vi "App - analyze RUS V6.vi"() -> ()   [LabVIEW 2021] (continued)
"file format"=enum."binary", "power(V)"=2.1, "Magn Field(T) "=0.0}, {"temperature"=14.639, "temperature str"="14.63900", "file path"=path "D:/Data/Ultrasound/LSCO/LSCO22__130814c/5_Cooling_2nd_try/September_2014/091814/14.63900K_500_2500_2.10000V_0.00000T_Sep18-2014__09-59-22_001_091814.bin", "last mod"=timestamp(3493893562 s since 1904-01-01), "file name str"="D:\\Data\\Ultrasound\\LSCO\\LSCO22__130814c\\5_Cooling_2nd_try\\September_2014\\091814\\14.63900K_500_2500_2.10000V_0.00000T_Sep18-2014__09-59-22_001_091814.bin", "mod time(min)"=58231559.36666667, "file format"=enum."binary", "power(V)"=2.1, "Magn Field(T) "=0.0}, {"temperature"=14.64, "temperature str"="14.64000", "file path"=path "D:/Data/Ultrasound/LSCO/LSCO22__130814c/5_Cooling_2nd_try/September_2014/091814/14.64000K_500_2500_2.10000V_0.00000T_Sep18-2014__10-00-41_001_091814.bin", "last mod"=timestamp(3493893641 s since 1904-01-01), "file name str"="D:\\Data\\Ultrasound\\LSCO\\LSCO22__130814c\\5_Cooling_2nd_try\\September_2014\\091814\\14.64000K_500_2500_2.10000V_0.00000T_Sep18-2014__10-00-41_001_091814.bin", "mod time(min)"=58231560.68333333, "file format"=enum."binary", "power(V)"=2.1, "Magn Field(T) "=0.0}, {"temperature"=14.641, "temperature str"="14.64100", "file path"=path "D:/Data/Ultrasound/LSCO/LSCO22__130814c/5_Cooling_2nd_try/September_2014/091814/14.64100K_500_2500_2.10000V_0.00000T_Sep18-2014__10-02-01_001_091814.bin", "last mod"=timestamp(3493893721 s since 1904-01-01), "file name str"="D:\\Data\\Ultrasound\\LSCO\\LSCO22__130814c\\5_Cooling_2nd_try\\September_2014\\091814\\14.64100K_500_2500_2.10000V_0.00000T_Sep18-2014__10-02-01_001_091814.bin", "mod time(min)"=58231562.016666666, "file format"=enum."binary", "power(V)"=2.1, "Magn Field(T) "=0.0}, {"temperature"=14.644, "temperature str"="14.64400", "file path"=path "D:/Data/Ultrasound/LSCO/LSCO22__130814c/5_Cooling_2nd_try/September_2014/091814/14.64400K_500_2500_2.10000V_0.00000T_Sep18-2014__10-03-20_001_091814.bin", "last mod"=timestamp(3493893800 s since 1904-01-01), "file name str"="D:\\Data\\Ultrasound\\LSCO\\LSCO22__130814c\\5_Cooling_2nd_try\\September_2014\\091814\\14.64400K_500_2500_2.10000V_0.00000T_Sep18-2014__10-03-20_001_091814.bin", "mod time(min)"=58231563.333333336, "file format"=enum."binary", "power(V)"=2.1, "Magn Field(T) "=0.0}, {"temperature"=14.65, "temperature str"="14.65000", "file path"=path "D:/Data/Ultrasound/LSCO/LSCO22__130814c/5_Cooling_2nd_try/September_2014/091814/14.65000K_500_2500_2.10000V_0.00000T_Sep18-2014__10-04-39_001_091814.bin", "last mod"=timestamp(3493893879 s since 1904-01-01), "file name str"="D:\\Data\\Ultrasound\\LSCO\\LSCO22__130814c\\5_Cooling_2nd_try\\September_2014\\091814\\14.65000K_500_2500_2.10000V_0.00000T_Sep18-2014__10-04-39_001_091814.bin", "mod time(min)"=58231564.65, "file format"=enum."binary", "power(V)"=2.1, "Magn Field(T) "=0.0}, {"temperature"=14.65, "temperature str"="14.65000", "file path"=path "D:/Data/Ultrasound/LSCO/LSCO22__130814c/5_Cooling_2nd_try/September_2014/091814/14.65000K_500_2500_2.10000V_0.00000T_Sep18-2014__10-05-59_001_091814.bin", "last mod"=timestamp(3493893959 s since 1904-01-01), "file name str"="D:\\Data\\Ultrasound\\LSCO\\LSCO22__130814c\\5_Cooling_2nd_try\\September_2014\\091814\\14.65000K_500_2500_2.10000V_0.00000T_Sep18-2014__10-05-59_001_091814.bin", "mod time(min)"=58231565.983333334, "file format"=enum."binary", "power(V)"=2.1, "Magn Field(T) "=0.0}, {"temperature"=14.654, "temperature str"="14.65400", "file path"=path "D:/Data/Ultrasound/LSCO/LSCO22__130814c/5_Cooling_2nd_try/September_2014/091814/14.65400K_500_2500_2.10000V_0.00000T_Sep18-2014__10-07-18_001_091814.bin", "last mod"=timestamp(3493894038 s since 1904-01-01), "file name str"="D:\\Data\\Ultrasound\\LSCO\\LSCO22__130814c\\5_Cooling_2nd_try\\September_2014\\091814\\14.65400K_500_2500_2.10000V_0.00000T_Sep18-2014__10-07-18_001_091814.bin", "mod time(min)"=58231567.3, "file format"=enum."binary", "power(V)"=2.1, "Magn Field(T) "=0.0}, {"temperature"=14.654, "temperature str"="14.65400", "file path"=path "D:/Data/Ultrasound/LSCO/LSCO22__130814c/5_Cooling_2nd_try/September_2014/091814/14.65400K_500_2500_2.10000V_0.00000T_Sep18-2014__10-08-38_001_091814.bin", "last mod"=timestamp(3493894118 s since 1904-01-01), "file name str"="D:\\Data\\Ultrasound\\LSCO\\LSCO22__130814c\\5_Cooling_2nd_try\\September_2014\\091814\\14.65400K_500_2500_2.10000V_0.00000T_Sep18-2014__10-08-38_001_091814.bin", "mod time(min)"=58231568.63333333, "file format"=enum."binary", "power(V)"=2.1, "Magn Field(T) "=0.0}, {"temperature"=14.657, "temperature str"="14.65700", "file path"=path "D:/Data/Ultrasound/LSCO/LSCO22__130814c/5_Cooling_2nd_try/September_2014/091814/14.65700K_500_2500_2.10000V_0.00000T_Sep18-2014__10-09-57_001_091814.bin", "last mod"=timestamp(3493894197 s since 1904-01-01), "file name str"="D:\\Data\\Ultrasound\\LSCO\\LSCO22__130814c\\5_Cooling_2nd_try\\September_2014\\091814\\14.65700K_500_2500_2.10000V_0.00000T_Sep18-2014__10-09-57_001_091814.bin", "mod time(min)"=58231569.95, "file format"=enum."binary", "power(V)"=2.1, "Magn Field(T) "=0.0}, {"temperature"=14.659, "temperature str"="14.65900", "file path"=path "D:/Data/Ultrasound/LSCO/LSCO22__130814c/5_Cooling_2nd_try/September_2014/091814/14.65900K_500_2500_2.10000V_0.00000T_Sep18-2014__10-11-16_001_091814.bin", "last mod"=timestamp(3493894276 s since 1904-01-01), "file name str"="D:\\Data\\Ultrasound\\LSCO\\LSCO22__130814c\\5_Cooling_2nd_try\\September_2014\\091814\\14.65900K_500_2500_2.10000V_0.00000T_Sep18-2014__10-11-16_001_091814.bin", "mod time(min)"=58231571.266666666, "file format"=enum."binary", "power(V)"=2.1, "Magn Field(T) "=0.0}, {"temperature"=14.66, "temperature str"="14.66000", "file path"=path "D:/Data/Ultrasound/LSCO/LSCO22__130814c/5_Cooling_2nd_try/September_2014/091814/14.66000K_500_2500_2.10000V_0.00000T_Sep18-2014__10-12-36_001_091814.bin", "last mod"=timestamp(3493894356 s since 1904-01-01), "file name str"="D:\\Data\\Ultrasound\\LSCO\\LSCO22__130814c\\5_Cooling_2nd_try\\September_2014\\091814\\14.66000K_500_2500_2.10000V_0.00000T_Sep18-2014__10-12-36_001_091814.bin", "mod time(min)"=58231572.6, "file format"=enum."binary", "power(V)"=2.1, "Magn Field(T) "=0.0}, {"temperature"=14.661, "temperature str"="14.66100", "file path"=path "D:/Data/Ultrasound/LSCO/LSCO22__130814c/5_Cooling_2nd_try/September_2014/091814/14.66100K_500_2500_2.10000V_0.00000T_Sep18-2014__10-13-55_001_091814.bin", "last mod"=timestamp(3493894435 s since 1904-01-01), "file name str"="D:\\Data\\Ultrasound\\LSCO\\LSCO22__130814c\\5_Cooling_2nd_try\\September_2014\\091814\\14.66100K_500_2500_2.10000V_0.00000T_Sep18-2014__10-13-55_001_091814.bin", "mod time(min)"=58231573.916666664, "file format"=enum."binary", "power(V)"=2.1, "Magn Field(T) "=0.0}, {"temperature"=14.664, "temperature str"="14.66400", "file path"=path "D:/Data/Ultrasound/LSCO/LSCO22__130814c/5_Cooling_2nd_try/September_2014/091814/14.66400K_500_2500_2.10000V_0.00000T_Sep18-2014__10-15-14_001_091814.bin", "last mod"=timestamp(3493894514 s since 1904-01-01), "file name str"="D:\\Data\\Ultrasound\\LSCO\\LSCO22__130814c\\5_Cooling_2nd_try\\September_2014\\091814\\14.66400K_500_2500_2.10000V_0.00000T_Sep18-2014__10-15-14_001_091814.bin", "mod time(min)"=58231575.233333334, "file format"=enum."binary", "power(V)"=2.1, "Magn Field(T) "=0.0}, {"temperature"=14.668, "temperature str"="14.66800", "file path"=path "D:/Data/Ultrasound/LSCO/LSCO22__130814c/5_Cooling_2nd_try/September_2014/091814/14.66800K_500_2500_2.10000V_0.00000T_Sep18-2014__10-16-34_001_091814.bin", "last mod"=timestamp(3493894594 s since 1904-01-01), "file name str"="D:\\Data\\Ultrasound\\LSCO\\LSCO22__130814c\\5_Cooling_2nd_try\\September_2014\\091814\\14.66800K_500_2500_2.10000V_0.00000T_Sep18-2014__10-16-34_001_091814.bin", "mod time(min)"=58231576.56666667, "file format"=enum."binary", "power(V)"=2.1, "Magn Field(T) "=0.0}, {"temperature"=14.669, "temperature str"="14.66900", "file path"=path "D:/Data/Ultrasound/LSCO/LSCO22__130814c/5_Cooling_2nd_try/September_2014/091814/14.66900K_500_2500_2.10000V_0.00000T_Sep18-2014__10-17-53_001_091814.bin", "last mod"=timestamp(3493894673 s since 1904-01-01), "file name str"="D:\\Data\\Ultrasound\\LSCO\\LSCO22__130814c\\5_Cooling_2nd_try\\September_2014\\091814\\14.66900K_500_2500_2.10000V_0.00000T_Sep18-2014__10-17-53_001_091814.bin", "mod time(min)"=58231577.88333333, "file format"=enum."binary", "power(V)"=2.1, "Magn Field(T) "=0.0}, {"temperature"=14.673, "temperature str"="14.67300", "file path"=path "D:/Data/Ultrasound/LSCO/LSCO22__130814c/5_Cooling_2nd_try/September_2014/091814/14.67300K_500_2500_2.10000V_0.00000T_Sep18-2014__10-19-13_001_091814.bin", "last mod"=timestamp(3493894753 s since 1904-01-01), "file name str"="D:\\Data\\Ultrasound\\LSCO\\LSCO22__130814c\\5_Cooling_2nd_try\\September_2014\\091814\\14.67300K_500_2500_2.10000V_0.00000T_Sep18-2014__10-19-13_001_091814.bin", "mod time(min)"=58231579.21666667, "file format"=enum."binary", "power(V)"=2.1, "Magn Field(T) "=0.0}, {"temperature"=14.673, "temperature str"="14.67300", "file path"=path "D:/Data/Ultrasound/LSCO/LSCO22__130814c/5_Cooling_2nd_try/September_2014/091814/14.67300K_500_2500_2.10000V_0.00000T_Sep18-2014__10-20-32_001_091814.bin", "last mod"=timestamp(3493894832 s since 1904-01-01), "file name str"="D:\\Data\\Ultrasound\\LSCO\\LSCO22__130814c\\5_Cooling_2nd_try\\September_2014\\091814\\14.67300K_500_2500_2.10000V_0.00000T_Sep18-2014__10-20-32_001_091814.bin", "mod time(min)"=58231580.53333333, "file format"=enum."binary", "power(V)"=2.1, "Magn Field(T) "=0.0}, {"temperature"=14.673, "temperature str"="14.67300", "file path"=path "D:/Data/Ultrasound/LSCO/LSCO22__130814c/5_Cooling_2nd_try/September_2014/091814/14.67300K_500_2500_2.10000V_0.00000T_Sep18-2014__10-21-51_001_091814.bin", "last mod"=timestamp(3493894911 s since 1904-01-01), "file name str"="D:\\Data\\Ultrasound\\LSCO\\LSCO22__130814c\\5_Cooling_2nd_try\\September_2014\\091814\\14.67300K_500_2500_2.10000V_0.00000T_Sep18-2014__10-21-51_001_091814.bin", "mod time(min)"=58231581.85, "file format"=enum."binary", "power(V)"=2.1, "Magn Field(T) "=0.0}, {"temperature"=14.676, "temperature str"="14.67600", "file path"=path "D:/Data/Ultrasound/LSCO/LSCO22__130814c/5_Cooling_2nd_try/September_2014/091814/14.67600K_500_2500_2.10000V_0.00000T_Sep18-2014__10-23-11_001_091814.bin", "last mod"=timestamp(3493894991 s since 1904-01-01), "file name str"="D:\\Data\\Ultrasound\\LSCO\\LSCO22__130814c\\5_Cooling_2nd_try\\September_2014\\091814\\14.67600K_500_2500_2.10000V_0.00000T_Sep18-2014__10-23-11_001_091814.bin", "mod time(min)"=58231583.18333333, "file format"=enum."binary", "power(V)"=2.1, "Magn Field(T) "=0.0}, {"temperature"=14.678, "temperature str"="14.67800", "file path"=path "D:/Data/Ultrasound/LSCO/LSCO22__130814c/5_Cooling_2nd_try/September_2014/091814/14.67800K_500_2500_2.10000V_0.00000T_Sep18-2014__10-24-30_001_091814.bin", "last mod"=timestamp(3493895070 s since 1904-01-01), "file name str"="D:\\Data\\Ultrasound\\LSCO\\LSCO22__130814c\\5_Cooling_2nd_try\\September_2014\\091814\\14.67800K_500_2500_2.10000V_0.00000T_Sep18-2014__10-24-30_001_091814.bin", "mod time(min)"=58231584.5, "file format"=enum."binary", "power(V)"=2.1, "Magn Field(T) "=0.0}, {"temperature"=14.678, "temperature str"="14.67800", "file path"=path "D:/Data/Ultrasound/LSCO/LSCO22__130814c/5_Cooling_2nd_try/September_2014/091814/14.67800K_500_2500_2.10000V_0.00000T_Sep18-2014__10-25-49_001_091814.bin", "last mod"=timestamp(3493895149 s since 1904-01-01), "file name str"="D:\\Data\\Ultrasound\\LSCO\\LSCO22__130814c\\5_Cooling_2nd_try\\September_2014\\091814\\14.67800K_500_2500_2.10000V_0.00000T_Sep18-2014__10-25-49_001_091814.bin", "mod time(min)"=58231585.81666667, "file format"=enum."binary", "power(V)"=2.1, "Magn Field(T) "=0.0}, {"temperature"=14.681, "temperature str"="14.68100", "file path"=path "D:/Data/Ultrasound/LSCO/LSCO22__130814c/5_Cooling_2nd_try/September_2014/091814/14.68100K_500_2500_2.10000V_0.00000T_Sep18-2014__10-27-09_001_091814.bin", "last mod"=timestamp(3493895229 s since 1904-01-01), "file name str"="D:\\Data\\Ultrasound\\LSCO\\LSCO22__130814c\\5_Cooling_2nd_try\\September_2014\\091814\\14.68100K_500_2500_2.10000V_0.00000T_Sep18-2014__10-27-09_001_091814.bin", "mod time(min)"=58231587.15, "file format"=enum."binary", "power(V)"=2.1, "Magn Field(T) "=0.0}, {"temperature"=14.682, "temperature str"="14.68200", "file path"=path "D:/Data/Ultrasound/LSCO/LSCO22__130814c/5_Cooling_2nd_try/September_2014/091814/14.68200K_500_2500_2.10000V_0.00000T_Sep18-2014__10-28-28_001_091814.bin", "last mod"=timestamp(3493895308 s since 1904-01-01), "file name str"="D:\\Data\\Ultrasound\\LSCO\\LSCO22__130814c\\5_Cooling_2nd_try\\September_2014\\091814\\14.68200K_500_2500_2.10000V_0.00000T_Sep18-2014__10-28-28_001_091814.bin", "mod time(min)"=58231588.46666667, "file format"=enum."binary", "power(V)"=2.1, "Magn Field(T) "=0.0}, {"temperature"=14.685, "temperature str"="14.68500", "file path"=path "D:/Data/Ultrasound/LSCO/LSCO22__130814c/5_Cooling_2nd_try/September_2014/091814/14.68500K_500_2500_2.10000V_0.00000T_Sep18-2014__10-29-48_001_091814.bin", "last mod"=timestamp(3493895388 s since 1904-01-01), "file name str"="D:\\Data\\Ultrasound\\LSCO\\LSCO22__130814c\\5_Cooling_2nd_try\\September_2014\\091814\\14.68500K_500_2500_2.10000V_0.00000T_Sep18-2014__10-29-48_001_091814.bin", "mod time(min)"=58231589.8, "file format"=enum."binary", "power(V)"=2.1, "Magn Field(T) "=0.0}, {"temperature"=14.689, "temperature str"="14.68900", "file path"=path "D:/Data/Ultrasound/LSCO/LSCO22__130814c/5_Cooling_2nd_try/September_2014/091814/14.68900K_500_2500_2.10000V_0.00000T_Sep18-2014__10-31-07_001_091814.bin", "last mod"=timestamp(3493895467 s since 1904-01-01), "file name str"="D:\\Data\\Ultrasound\\LSCO\\LSCO22__130814c\\5_Cooling_2nd_try\\September_2014\\091814\\14.68900K_500_2500_2.10000V_0.00000T_Sep18-2014__10-31-07_001_091814.bin", "mod time(min)"=58231591.11666667, "file format"=enum."binary", "power(V)"=2.1, "Magn Field(T) "=0.0}, {"temperature"=14.687, "temperature str"="14.68700", "file path"=path "D:/Data/Ultrasound/LSCO/LSCO22__130814c/5_Cooling_2nd_try/September_2014/091814/14.68700K_500_2500_2.10000V_0.00000T_Sep18-2014__10-32-26_001_091814.bin", "last mod"=timestamp(3493895546 s since 1904-01-01), "file name str"="D:\\Data\\Ultrasound\\LSCO\\LSCO22__130814c\\5_Cooling_2nd_try\\September_2014\\091814\\14.68700K_500_2500_2.10000V_0.00000T_Sep18-2014__10-32-26_001_091814.bin", "mod time(min)"=58231592.43333333, "file format"=enum."binary", "power(V)"=2.1, "Magn Field(T) "=0.0}, {"temperature"=14.688, "temperature str"="14.68800", "file path"=path "D:/Data/Ultrasound/LSCO/LSCO22__130814c/5_Cooling_2nd_try/September_2014/091814/14.68800K_500_2500_2.10000V_0.00000T_Sep18-2014__10-33-46_001_091814.bin", "last mod"=timestamp(3493895626 s since 1904-01-01), "file name str"="D:\\Data\\Ultrasound\\LSCO\\LSCO22__130814c\\5_Cooling_2nd_try\\September_2014\\091814\\14.68800K_500_2500_2.10000V_0.00000T_Sep18-2014__10-33-46_001_091814.bin", "mod time(min)"=58231593.766666666, "file format"=enum."binary", "power(V)"=2.1, "Magn Field(T) "=0.0}, {"temperature"=14.693, "temperature str"="14.69300", "file path"=path "D:/Data/Ultrasound/LSCO/LSCO22__130814c/5_Cooling_2nd_try/September_2014/091814/14.69300K_500_2500_2.10000V_0.00000T_Sep18-2014__10-35-05_001_091814.bin", "last mod"=timestamp(3493895705 s since 1904-01-01), "file name str"="D:\\Data\\Ultrasound\\LSCO\\LSCO22__130814c\\5_Cooling_2nd_try\\September_2014\\091814\\14.69300K_500_2500_2.10000V_0.00000T_Sep18-2014__10-35-05_001_091814.bin", "mod time(min)"=58231595.083333336, "file format"=enum."binary", "power(V)"=2.1, "Magn Field(T) "=0.0}, {"temperature"=14.693, "temperature str"="14.69300", "file path"=path "D:/Data/Ultrasound/LSCO/LSCO22__130814c/5_Cooling_2nd_try/September_2014/091814/14.69300K_500_2500_2.10000V_0.00000T_Sep18-2014__10-36-24_001_091814.bin", "last mod"=timestamp(3493895784 s since 1904-01-01), "file name str"="D:\\Data\\Ultrasound\\LSCO\\LSCO22__130814c\\5_Cooling_2nd_try\\September_2014\\091814\\14.69300K_500_2500_2.10000V_0.00000T_Sep18-2014__10-36-24_001_091814.bin", "mod time(min)"=58231596.4, "file format"=enum."binary", "power(V)"=2.1, "Magn Field(T) "=0.0}, {"temperature"=14.696, "temperature str"="14.69600", "file path"=path "D:/Data/Ultrasound/LSCO/LSCO22__130814c/5_Cooling_2nd_try/September_2014/091814/14.69600K_500_2500_2.10000V_0.00000T_Sep18-2014__10-37-44_001_091814.bin", "last mod"=timestamp(3493895864 s since 1904-01-01), "file name str"="D:\\Data\\Ultrasound\\LSCO\\LSCO22__130814c\\5_Cooling_2nd_try\\September_2014\\091814\\14.69600K_500_2500_2.10000V_0.00000T_Sep18-2014__10-37-44_001_091814.bin", "mod time(min)"=58231597.733333334, "file format"=enum."binary", "power(V)"=2.1, "Magn Field(T) "=0.0}, {"temperature"=14.697, "temperature str"="14.69700", "file path"=path "D:/Data/Ultrasound/LSCO/LSCO22__130814c/5_Cooling_2nd_try/September_2014/091814/14.69700K_500_2500_2.10000V_0.00000T_Sep18-2014__10-39-03_001_091814.bin", "last mod"=timestamp(3493895943 s since 1904-01-01), "file name str"="D:\\Data\\Ultrasound\\LSCO\\LSCO22__130814c\\5_Cooling_2nd_try\\September_2014\\091814\\14.69700K_500_2500_2.10000V_0.00000T_Sep18-2014__10-39-03_001_091814.bin", "mod time(min)"=58231599.05, "file format"=enum."binary", "power(V)"=2.1, "Magn Field(T) "=0.0}, {"temperature"=14.697, "temperature str"="14.69700", "file path"=path "D:/Data/Ultrasound/LSCO/LSCO22__130814c/5_Cooling_2nd_try/September_2014/091814/14.69700K_500_2500_2.10000V_0.00000T_Sep18-2014__10-40-23_001_091814.bin", "last mod"=timestamp(3493896023 s since 1904-01-01), "file name str"="D:\\Data\\Ultrasound\\LSCO\\LSCO22__130814c\\5_Cooling_2nd_try\\September_2014\\091814\\14.69700K_500_2500_2.10000V_0.00000T_Sep18-2014__10-40-23_001_091814.bin", "mod time(min)"=58231600.38333333, "file format"=enum."binary", "power(V)"=2.1, "Magn Field(T) "=0.0}, {"temperature"=14.699, "temperature str"="14.69900", "file path"=path "D:/Data/Ultrasound/LSCO/LSCO22__130814c/5_Cooling_2nd_try/September_2014/091814/14.69900K_500_2500_2.10000V_0.00000T_Sep18-2014__10-41-42_001_091814.bin", "last mod"=timestamp(3493896102 s since 1904-01-01), "file name str"="D:\\Data\\Ultrasound\\LSCO\\LSCO22__130814c\\5_Cooling_2nd_try\\September_2014\\091814\\14.69900K_500_2500_2.10000V_0.00000T_Sep18-2014__10-41-42_001_091814.bin", "mod time(min)"=58231601.7, "file format"=enum."binary", "power(V)"=2.1, "Magn Field(T) "=0.0}, {"temperature"=14.702, "temperature str"="14.70200", "file path"=path "D:/Data/Ultrasound/LSCO/LSCO22__130814c/5_Cooling_2nd_try/September_2014/091814/14.70200K_500_2500_2.10000V_0.00000T_Sep18-2014__10-43-01_001_091814.bin", "last mod"=timestamp(3493896181 s since 1904-01-01), "file name str"="D:\\Data\\Ultrasound\\LSCO\\LSCO22__130814c\\5_Cooling_2nd_try\\September_2014\\091814\\14.70200K_500_2500_2.10000V_0.00000T_Sep18-2014__10-43-01_001_091814.bin", "mod time(min)"=58231603.016666666, "file format"=enum."binary", "power(V)"=2.1, "Magn Field(T) "=0.0}, {"temperature"=14.706, "temperature str"="14.70600", "file path"=path "D:/Data/Ultrasound/LSCO/LSCO22__130814c/5_Cooling_2nd_try/September_2014/091814/14.70600K_500_2500_2.10000V_0.00000T_Sep18-2014__10-44-21_001_091814.bin", "last mod"=timestamp(3493896261 s since 1904-01-01), "file name str"="D:\\Data\\Ultrasound\\LSCO\\LSCO22__130814c\\5_Cooling_2nd_try\\September_2014\\091814\\14.70600K_500_2500_2.10000V_0.00000T_Sep18-2014__10-44-21_001_091814.bin", "mod time(min)"=58231604.35, "file format"=enum."binary", "power(V)"=2.1, "Magn Field(T) "=0.0}, {"temperature"=14.708, "temperature str"="14.70800", "file path"=path "D:/Data/Ultrasound/LSCO/LSCO22__130814c/5_Cooling_2nd_try/September_2014/091814/14.70800K_500_2500_2.10000V_0.00000T_Sep18-2014__10-45-40_001_091814.bin", "last mod"=timestamp(3493896340 s since 1904-01-01), "file name str"="D:\\Data\\Ultrasound\\LSCO\\LSCO22__130814c\\5_Cooling_2nd_try\\September_2014\\091814\\14.70800K_500_2500_2.10000V_0.00000T_Sep18-2014__10-45-40_001_091814.bin", "mod time(min)"=58231605.666666664, "file format"=enum."binary", "power(V)"=2.1, "Magn Field(T) "=0.0}, {"temperature"=14.703, "temperature str"="14.70300", "file path"=path "D:/Data/Ultrasound/LSCO/LSCO22__130814c/5_Cooling_2nd_try/September_2014/091814/14.70300K_500_2500_2.10000V_0.00000T_Sep18-2014__10-46-59_001_091814.bin", "last mod"=timestamp(3493896419 s since 1904-01-01), "file name str"="D:\\Data\\Ultrasound\\LSCO\\LSCO22__130814c\\5_Cooling_2nd_try\\September_2014\\091814\\14.70300K_500_2500_2.10000V_0.00000T_Sep18-2014__10-46-59_001_091814.bin", "mod time(min)"=58231606.983333334, "file format"=enum."binary", "power(V)"=2.1, "Magn Field(T) "=0.0}, {"temperature"=14.705, "temperature str"="14.70500", "file path"=path "D:/Data/Ultrasound/LSCO/LSCO22__130814c/5_Cooling_2nd_try/September_2014/091814/14.70500K_500_2500_2.10000V_0.00000T_Sep18-2014__10-48-19_001_091814.bin", "last mod"=timestamp(3493896499 s since 1904-01-01), "file name str"="D:\\Data\\Ultrasound\\LSCO\\LSCO22__130814c\\5_Cooling_2nd_try\\September_2014\\091814\\14.70500K_500_2500_2.10000V_0.00000T_Sep18-2014__10-48-19_001_091814.bin", "mod time(min)"=58231608.31666667, "file format"=enum."binary", "power(V)"=2.1, "Magn Field(T) "=0.0}, {"temperature"=14.708, "temperature str"="14.70800", "file path"=path "D:/Data/Ultrasound/LSCO/LSCO22__130814c/5_Cooling_2nd_try/September_2014/091814/14.70800K_500_2500_2.10000V_0.00000T_Sep18-2014__10-49-38_001_091814.bin", "last mod"=timestamp(3493896578 s since 1904-01-01), "file name str"="D:\\Data\\Ultrasound\\LSCO\\LSCO22__130814c\\5_Cooling_2nd_try\\September_2014\\091814\\14.70800K_500_2500_2.10000V_0.00000T_Sep18-2014__10-49-38_001_091814.bin", "mod time(min)"=58231609.63333333, "file format"=enum."binary", "power(V)"=2.1, "Magn Field(T) "=0.0}, {"temperature"=14.709, "temperature str"="14.70900", "file path"=path "D:/Data/Ultrasound/LSCO/LSCO22__130814c/5_Cooling_2nd_try/September_2014/091814/14.70900K_500_2500_2.10000V_0.00000T_Sep18-2014__10-50-58_001_091814.bin", "last mod"=timestamp(3493896658 s since 1904-01-01), "file name str"="D:\\Data\\Ultrasound\\LSCO\\LSCO22__130814c\\5_Cooling_2nd_try\\September_2014\\091814\\14.70900K_500_2500_2.10000V_0.00000T_Sep18-2014__10-50-58_001_091814.bin", "mod time(min)"=58231610.96666667, "file format"=enum."binary", "power(V)"=2.1, "Magn Field(T) "=0.0}, {"temperature"=14.714, "temperature str"="14.71400", "file path"=path "D:/Data/Ultrasound/LSCO/LSCO22__130814c/5_Cooling_2nd_try/September_2014/091814/14.71400K_500_2500_2.10000V_0.00000T_Sep18-2014__10-52-17_001_091814.bin", "last mod"=timestamp(3493896737 s since 1904-01-01), "file name str"="D:\\Data\\Ultrasound\\LSCO\\LSCO22__130814c\\5_Cooling_2nd_try\\September_2014\\091814\\14.71400K_500_2500_2.10000V_0.00000T_Sep18-2014__10-52-17_001_091814.bin", "mod time(min)"=58231612.28333333, "file format"=enum."binary", "power(V)"=2.1, "Magn Field(T) "=0.0}, {"temperature"=14.719, "temperature str"="14.71900", "file path"=path "D:/Data/Ultrasound/LSCO/LSCO22__130814c/5_Cooling_2nd_try/September_2014/091814/14.71900K_500_2500_2.10000V_0.00000T_Sep18-2014__10-53-36_001_091814.bin", "last mod"=timestamp(3493896816 s since 1904-01-01), "file name str"="D:\\Data\\Ultrasound\\LSCO\\LSCO22__130814c\\5_Cooling_2nd_try\\September_2014\\091814\\14.71900K_500_2500_2.10000V_0.00000T_Sep18-2014__10-53-36_001_091814.bin", "mod time(min)"=58231613.6, "file format"=enum."binary", "power(V)"=2.1, "Magn Field(T) "=0.0}, {"temperature"=14.717, "temperature str"="14.71700", "file path"=path "D:/Data/Ultrasound/LSCO/LSCO22__130814c/5_Cooling_2nd_try/September_2014/091814/14.71700K_500_2500_2.10000V_0.00000T_Sep18-2014__10-54-56_001_091814.bin", "last mod"=timestamp(3493896896 s since 1904-01-01), "file name str"="D:\\Data\\Ultrasound\\LSCO\\LSCO22__130814c\\5_Cooling_2nd_try\\September_2014\\091814\\14.71700K_500_2500_2.10000V_0.00000T_Sep18-2014__10-54-56_001_091814.bin", "mod time(min)"=58231614.93333333, "file format"=enum."binary", "power(V)"=2.1, "Magn Field(T) "=0.0}, {"temperature"=14.723, "temperature str"="14.72300", "file path"=path "D:/Data/Ultrasound/LSCO/LSCO22__130814c/5_Cooling_2nd_try/September_2014/091814/14.72300K_500_2500_2.10000V_0.00000T_Sep18-2014__10-56-15_001_091814.bin", "last mod"=timestamp(3493896975 s since 1904-01-01), "file name str"="D:\\Data\\Ultrasound\\LSCO\\LSCO22__130814c\\5_Cooling_2nd_try\\September_2014\\091814\\14.72300K_500_2500_2.10000V_0.00000T_Sep18-2014__10-56-15_001_091814.bin", "mod time(min)"=58231616.25, "file format"=enum."binary", "power(V)"=2.1, "Magn Field(T) "=0.0}, {"temperature"=14.725, "temperature str"="14.72500", "file path"=path "D:/Data/Ultrasound/LSCO/LSCO22__130814c/5_Cooling_2nd_try/September_2014/091814/14.72500K_500_2500_2.10000V_0.00000T_Sep18-2014__10-57-34_001_091814.bin", "last mod"=timestamp(3493897054 s since 1904-01-01), "file name str"="D:\\Data\\Ultrasound\\LSCO\\LSCO22__130814c\\5_Cooling_2nd_try\\September_2014\\091814\\14.72500K_500_2500_2.10000V_0.00000T_Sep18-2014__10-57-34_001_091814.bin", "mod time(min)"=58231617.56666667, "file format"=enum."binary", "power(V)"=2.1, "Magn Field(T) "=0.0}, {"temperature"=14.727, "temperature str"="14.72700", "file path"=path "D:/Data/Ultrasound/LSCO/LSCO22__130814c/5_Cooling_2nd_try/September_2014/091814/14.72700K_500_2500_2.10000V_0.00000T_Sep18-2014__10-58-54_001_091814.bin", "last mod"=timestamp(3493897134 s since 1904-01-01), "file name str"="D:\\Data\\Ultrasound\\LSCO\\LSCO22__130814c\\5_Cooling_2nd_try\\September_2014\\091814\\14.72700K_500_2500_2.10000V_0.00000T_Sep18-2014__10-58-54_001_091814.bin", "mod time(min)"=58231618.9, "file format"=enum."binary", "power(V)"=2.1, "Magn Field(T) "=0.0}, {"temperature"=14.732, "temperature str"="14.73200", "file path"=path "D:/Data/Ultrasound/LSCO/LSCO22__130814c/5_Cooling_2nd_try/September_2014/091814/14.73200K_500_2500_2.10000V_0.00000T_Sep18-2014__11-00-13_001_091814.bin", "last mod"=timestamp(3493897213 s since 1904-01-01), "file name str"="D:\\Data\\Ultrasound\\LSCO\\LSCO22__130814c\\5_Cooling_2nd_try\\September_2014\\091814\\14.73200K_500_2500_2.10000V_0.00000T_Sep18-2014__11-00-13_001_091814.bin", "mod time(min)"=58231620.21666667, "file format"=enum."binary", "power(V)"=2.1, "Magn Field(T) "=0.0}, {"temperature"=14.737, "temperature str"="14.73700", "file path"=path "D:/Data/Ultrasound/LSCO/LSCO22__130814c/5_Cooling_2nd_try/September_2014/091814/14.73700K_500_2500_2.10000V_0.00000T_Sep18-2014__11-01-33_001_091814.bin", "last mod"=timestamp(3493897293 s since 1904-01-01), "file name str"="D:\\Data\\Ultrasound\\LSCO\\LSCO22__130814c\\5_Cooling_2nd_try\\September_2014\\091814\\14.73700K_500_2500_2.10000V_0.00000T_Sep18-2014__11-01-33_001_091814.bin", "mod time(min)"=58231621.55, "file format"=enum."binary", "power(V)"=2.1, "Magn Field(T) "=0.0}, {"temperature"=14.737, "temperature str"="14.73700", "file path"=path "D:/Data/Ultrasound/LSCO/LSCO22__130814c/5_Cooling_2nd_try/September_2014/091814/14.73700K_500_2500_2.10000V_0.00000T_Sep18-2014__11-02-52_001_091814.bin", "last mod"=timestamp(3493897372 s since 1904-01-01), "file name str"="D:\\Data\\Ultrasound\\LSCO\\LSCO22__130814c\\5_Cooling_2nd_try\\September_2014\\091814\\14.73700K_500_2500_2.10000V_0.00000T_Sep18-2014__11-02-52_001_091814.bin", "mod time(min)"=58231622.86666667, "file format"=enum."binary", "power(V)"=2.1, "Magn Field(T) "=0.0}, {"temperature"=14.739, "temperature str"="14.73900", "file path"=path "D:/Data/Ultrasound/LSCO/LSCO22__130814c/5_Cooling_2nd_try/September_2014/091814/14.73900K_500_2500_2.10000V_0.00000T_Sep18-2014__11-04-11_001_091814.bin", "last mod"=timestamp(3493897451 s since 1904-01-01), "file name str"="D:\\Data\\Ultrasound\\LSCO\\LSCO22__130814c\\5_Cooling_2nd_try\\September_2014\\091814\\14.73900K_500_2500_2.10000V_0.00000T_Sep18-2014__11-04-11_001_091814.bin", "mod time(min)"=58231624.18333333, "file format"=enum."binary", "power(V)"=2.1, "Magn Field(T) "=0.0}, {"temperature"=14.744, "temperature str"="14.74400", "file path"=path "D:/Data/Ultrasound/LSCO/LSCO22__130814c/5_Cooling_2nd_try/September_2014/091814/14.74400K_500_2500_2.10000V_0.00000T_Sep18-2014__11-05-31_001_091814.bin", "last mod"=timestamp(3493897531 s since 1904-01-01), "file name str"="D:\\Data\\Ultrasound\\LSCO\\LSCO22__130814c\\5_Cooling_2nd_try\\September_2014\\091814\\14.74400K_500_2500_2.10000V_0.00000T_Sep18-2014__11-05-31_001_091814.bin", "mod time(min)"=58231625.516666666, "file format"=enum."binary", "power(V)"=2.1, "Magn Field(T) "=0.0}, {"temperature"=14.747, "temperature str"="14.74700", "file path"=path "D:/Data/Ultrasound/LSCO/LSCO22__130814c/5_Cooling_2nd_try/September_2014/091814/14.74700K_500_2500_2.10000V_0.00000T_Sep18-2014__11-06-50_001_091814.bin", "last mod"=timestamp(3493897610 s since 1904-01-01), "file name str"="D:\\Data\\Ultrasound\\LSCO\\LSCO22__130814c\\5_Cooling_2nd_try\\September_2014\\091814\\14.74700K_500_2500_2.10000V_0.00000T_Sep18-2014__11-06-50_001_091814.bin", "mod time(min)"=58231626.833333336, "file format"=enum."binary", "power(V)"=2.1, "Magn Field(T) "=0.0}, {"temperature"=14.75, "temperature str"="14.75000", "file path"=path "D:/Data/Ultrasound/LSCO/LSCO22__130814c/5_Cooling_2nd_try/September_2014/091814/14.75000K_500_2500_2.10000V_0.00000T_Sep18-2014__11-08-09_001_091814.bin", "last mod"=timestamp(3493897689 s since 1904-01-01), "file name str"="D:\\Data\\Ultrasound\\LSCO\\LSCO22__130814c\\5_Cooling_2nd_try\\September_2014\\091814\\14.75000K_500_2500_2.10000V_0.00000T_Sep18-2014__11-08-09_001_091814.bin", "mod time(min)"=58231628.15, "file format"=enum."binary", "power(V)"=2.1, "Magn Field(T) "=0.0}, {"temperature"=14.751, "temperature str"="14.75100", "file path"=path "D:/Data/Ultrasound/LSCO/LSCO22__130814c/5_Cooling_2nd_try/September_2014/091814/14.75100K_500_2500_2.10000V_0.00000T_Sep18-2014__11-09-29_001_091814.bin", "last mod"=timestamp(3493897769 s since 1904-01-01), "file name str"="D:\\Data\\Ultrasound\\LSCO\\LSCO22__130814c\\5_Cooling_2nd_try\\September_2014\\091814\\14.75100K_500_2500_2.10000V_0.00000T_Sep18-2014__11-09-29_001_091814.bin", "mod time(min)"=58231629.483333334, "file format"=enum."binary", "power(V)"=2.1, "Magn Field(T) "=0.0}, {"temperature"=14.757, "temperature str"="14.75700", "file path"=path "D:/Data/Ultrasound/LSCO/LSCO22__130814c/5_Cooling_2nd_try/September_2014/091814/14.75700K_500_2500_2.10000V_0.00000T_Sep18-2014__11-10-48_001_091814.bin", "last mod"=timestamp(3493897848 s since 1904-01-01), "file name str"="D:\\Data\\Ultrasound\\LSCO\\LSCO22__130814c\\5_Cooling_2nd_try\\September_2014\\091814\\14.75700K_500_2500_2.10000V_0.00000T_Sep18-2014__11-10-48_001_091814.bin", "mod time(min)"=58231630.8, "file format"=enum."binary", "power(V)"=2.1, "Magn Field(T) "=0.0}, {"temperature"=14.754, "temperature str"="14.75400", "file path"=path "D:/Data/Ultrasound/LSCO/LSCO22__130814c/5_Cooling_2nd_try/September_2014/091814/14.75400K_500_2500_2.10000V_0.00000T_Sep18-2014__11-12-08_001_091814.bin", "last mod"=timestamp(3493897928 s since 1904-01-01), "file name str"="D:\\Data\\Ultrasound\\LSCO\\LSCO22__130814c\\5_Cooling_2nd_try\\September_2014\\091814\\14.75400K_500_2500_2.10000V_0.00000T_Sep18-2014__11-12-08_001_091814.bin", "mod time(min)"=58231632.13333333, "file format"=enum."binary", "power(V)"=2.1, "Magn Field(T) "=0.0}, {"temperature"=14.762, "temperature str"="14.76200", "file path"=path "D:/Data/Ultrasound/LSCO/LSCO22__130814c/5_Cooling_2nd_try/September_2014/091814/14.76200K_500_2500_2.10000V_0.00000T_Sep18-2014__11-13-27_001_091814.bin", "last mod"=timestamp(3493898007 s since 1904-01-01), "file name str"="D:\\Data\\Ultrasound\\LSCO\\LSCO22__130814c\\5_Cooling_2nd_try\\September_2014\\091814\\14.76200K_500_2500_2.10000V_0.00000T_Sep18-2014__11-13-27_001_091814.bin", "mod time(min)"=58231633.45, "file format"=enum."binary", "power(V)"=2.1, "Magn Field(T) "=0.0}, {"temperature"=14.757, "temperature str"="14.75700", "file path"=path "D:/Data/Ultrasound/LSCO/LSCO22__130814c/5_Cooling_2nd_try/September_2014/091814/14.75700K_500_2500_2.10000V_0.00000T_Sep18-2014__11-14-46_001_091814.bin", "last mod"=timestamp(3493898086 s since 1904-01-01), "file name str"="D:\\Data\\Ultrasound\\LSCO\\LSCO22__130814c\\5_Cooling_2nd_try\\September_2014\\091814\\14.75700K_500_2500_2.10000V_0.00000T_Sep18-2014__11-14-46_001_091814.bin", "mod time(min)"=58231634.766666666, "file format"=enum."binary", "power(V)"=2.1, "Magn Field(T) "=0.0}, {"temperature"=14.761, "temperature str"="14.76100", "file path"=path "D:/Data/Ultrasound/LSCO/LSCO22__130814c/5_Cooling_2nd_try/September_2014/091814/14.76100K_500_2500_2.10000V_0.00000T_Sep18-2014__11-16-06_001_091814.bin", "last mod"=timestamp(3493898166 s since 1904-01-01), "file name str"="D:\\Data\\Ultrasound\\LSCO\\LSCO22__130814c\\5_Cooling_2nd_try\\September_2014\\091814\\14.76100K_500_2500_2.10000V_0.00000T_Sep18-2014__11-16-06_001_091814.bin", "mod time(min)"=58231636.1, "file format"=enum."binary", "power(V)"=2.1, "Magn Field(T) "=0.0}, {"temperature"=14.768, "temperature str"="14.76800", "file path"=path "D:/Data/Ultrasound/LSCO/LSCO22__130814c/5_Cooling_2nd_try/September_2014/091814/14.76800K_500_2500_2.10000V_0.00000T_Sep18-2014__11-17-25_001_091814.bin", "last mod"=timestamp(3493898245 s since 1904-01-01), "file name str"="D:\\Data\\Ultrasound\\LSCO\\LSCO22__130814c\\5_Cooling_2nd_try\\September_2014\\091814\\14.76800K_500_2500_2.10000V_0.00000T_Sep18-2014__11-17-25_001_091814.bin", "mod time(min)"=58231637.416666664, "file format"=enum."binary", "power(V)"=2.1, "Magn Field(T) "=0.0}, {"temperature"=14.764, "temperature str"="14.76400", "file path"=path "D:/Data/Ultrasound/LSCO/LSCO22__130814c/5_Cooling_2nd_try/September_2014/091814/14.76400K_500_2500_2.10000V_0.00000T_Sep18-2014__11-18-44_001_091814.bin", "last mod"=timestamp(3493898324 s since 1904-01-01), "file name str"="D:\\Data\\Ultrasound\\LSCO\\LSCO22__130814c\\5_Cooling_2nd_try\\September_2014\\091814\\14.76400K_500_2500_2.10000V_0.00000T_Sep18-2014__11-18-44_001_091814.bin", "mod time(min)"=58231638.733333334, "file format"=enum."binary", "power(V)"=2.1, "Magn Field(T) "=0.0}, {"temperature"=14.769, "temperature str"="14.76900", "file path"=path "D:/Data/Ultrasound/LSCO/LSCO22__130814c/5_Cooling_2nd_try/September_2014/091814/14.76900K_500_2500_2.10000V_0.00000T_Sep18-2014__11-20-04_001_091814.bin", "last mod"=timestamp(3493898404 s since 1904-01-01), "file name str"="D:\\Data\\Ultrasound\\LSCO\\LSCO22__130814c\\5_Cooling_2nd_try\\September_2014\\091814\\14.76900K_500_2500_2.10000V_0.00000T_Sep18-2014__11-20-04_001_091814.bin", "mod time(min)"=58231640.06666667, "file format"=enum."binary", "power(V)"=2.1, "Magn Field(T) "=0.0}, {"temperature"=14.773, "temperature str"="14.77300", "file path"=path "D:/Data/Ultrasound/LSCO/LSCO22__130814c/5_Cooling_2nd_try/September_2014/091814/14.77300K_500_2500_2.10000V_0.00000T_Sep18-2014__11-21-23_001_091814.bin", "last mod"=timestamp(3493898483 s since 1904-01-01), "file name str"="D:\\Data\\Ultrasound\\LSCO\\LSCO22__130814c\\5_Cooling_2nd_try\\September_2014\\091814\\14.77300K_500_2500_2.10000V_0.00000T_Sep18-2014__11-21-23_001_091814.bin", "mod time(min)"=58231641.38333333, "file format"=enum."binary", "power(V)"=2.1, "Magn Field(T) "=0.0}, {"temperature"=14.772, "temperature str"="14.77200", "file path"=path "D:/Data/Ultrasound/LSCO/LSCO22__130814c/5_Cooling_2nd_try/September_2014/091814/14.77200K_500_2500_2.10000V_0.00000T_Sep18-2014__11-22-43_001_091814.bin", "last mod"=timestamp(3493898563 s since 1904-01-01), "file name str"="D:\\Data\\Ultrasound\\LSCO\\LSCO22__130814c\\5_Cooling_2nd_try\\September_2014\\091814\\14.77200K_500_2500_2.10000V_0.00000T_Sep18-2014__11-22-43_001_091814.bin", "mod time(min)"=58231642.71666667, "file format"=enum."binary", "power(V)"=2.1, "Magn Field(T) "=0.0}, {"temperature"=14.778, "temperature str"="14.77800", "file path"=path "D:/Data/Ultrasound/LSCO/LSCO22__130814c/5_Cooling_2nd_try/September_2014/091814/14.77800K_500_2500_2.10000V_0.00000T_Sep18-2014__11-24-02_001_091814.bin", "last mod"=timestamp(3493898642 s since 1904-01-01), "file name str"="D:\\Data\\Ultrasound\\LSCO\\LSCO22__130814c\\5_Cooling_2nd_try\\September_2014\\091814\\14.77800K_500_2500_2.10000V_0.00000T_Sep18-2014__11-24-02_001_091814.bin", "mod time(min)"=58231644.03333333, "file format"=enum."binary", "power(V)"=2.1, "Magn Field(T) "=0.0}, {"temperature"=14.778, "temperature str"="14.77800", "file path"=path "D:/Data/Ultrasound/LSCO/LSCO22__130814c/5_Cooling_2nd_try/September_2014/091814/14.77800K_500_2500_2.10000V_0.00000T_Sep18-2014__11-25-21_001_091814.bin", "last mod"=timestamp(3493898721 s since 1904-01-01), "file name str"="D:\\Data\\Ultrasound\\LSCO\\LSCO22__130814c\\5_Cooling_2nd_try\\September_2014\\091814\\14.77800K_500_2500_2.10000V_0.00000T_Sep18-2014__11-25-21_001_091814.bin", "mod time(min)"=58231645.35, "file format"=enum."binary", "power(V)"=2.1, "Magn Field(T) "=0.0}, {"temperature"=14.778, "temperature str"="14.77800", "file path"=path "D:/Data/Ultrasound/LSCO/LSCO22__130814c/5_Cooling_2nd_try/September_2014/091814/14.77800K_500_2500_2.10000V_0.00000T_Sep18-2014__11-26-41_001_091814.bin", "last mod"=timestamp(3493898801 s since 1904-01-01), "file name str"="D:\\Data\\Ultrasound\\LSCO\\LSCO22__130814c\\5_Cooling_2nd_try\\September_2014\\091814\\14.77800K_500_2500_2.10000V_0.00000T_Sep18-2014__11-26-41_001_091814.bin", "mod time(min)"=58231646.68333333, "file format"=enum."binary", "power(V)"=2.1, "Magn Field(T) "=0.0}, {"temperature"=14.784, "temperature str"="14.78400", "file path"=path "D:/Data/Ultrasound/LSCO/LSCO22__130814c/5_Cooling_2nd_try/September_2014/091814/14.78400K_500_2500_2.10000V_0.00000T_Sep18-2014__11-28-00_001_091814.bin", "last mod"=timestamp(3493898880 s since 1904-01-01), "file name str"="D:\\Data\\Ultrasound\\LSCO\\LSCO22__130814c\\5_Cooling_2nd_try\\September_2014\\091814\\14.78400K_500_2500_2.10000V_0.00000T_Sep18-2014__11-28-00_001_091814.bin", "mod time(min)"=58231648.0, "file format"=enum."binary", "power(V)"=2.1, "Magn Field(T) "=0.0}, {"temperature"=14.784, "temperature str"="14.78400", "file path"=path "D:/Data/Ultrasound/LSCO/LSCO22__130814c/5_Cooling_2nd_try/September_2014/091814/14.78400K_500_2500_2.10000V_0.00000T_Sep18-2014__11-29-19_001_091814.bin", "last mod"=timestamp(3493898959 s since 1904-01-01), "file name str"="D:\\Data\\Ultrasound\\LSCO\\LSCO22__130814c\\5_Cooling_2nd_try\\September_2014\\091814\\14.78400K_500_2500_2.10000V_0.00000T_Sep18-2014__11-29-19_001_091814.bin", "mod time(min)"=58231649.31666667, "file format"=enum."binary", "power(V)"=2.1, "Magn Field(T) "=0.0}, {"temperature"=14.784, "temperature str"="14.78400", "file path"=path "D:/Data/Ultrasound/LSCO/LSCO22__130814c/5_Cooling_2nd_try/September_2014/091814/14.78400K_500_2500_2.10000V_0.00000T_Sep18-2014__11-30-39_001_091814.bin", "last mod"=timestamp(3493899039 s since 1904-01-01), "file name str"="D:\\Data\\Ultrasound\\LSCO\\LSCO22__130814c\\5_Cooling_2nd_try\\September_2014\\091814\\14.78400K_500_2500_2.10000V_0.00000T_Sep18-2014__11-30-39_001_091814.bin", "mod time(min)"=58231650.65, "file format"=enum."binary", "power(V)"=2.1, "Magn Field(T) "=0.0}, {"temperature"=14.789, "temperature str"="14.78900", "file path"=path "D:/Data/Ultrasound/LSCO/LSCO22__130814c/5_Cooling_2nd_try/September_2014/091814/14.78900K_500_2500_2.10000V_0.00000T_Sep18-2014__11-31-58_001_091814.bin", "last mod"=timestamp(3493899118 s since 1904-01-01), "file name str"="D:\\Data\\Ultrasound\\LSCO\\LSCO22__130814c\\5_Cooling_2nd_try\\September_2014\\091814\\14.78900K_500_2500_2.10000V_0.00000T_Sep18-2014__11-31-58_001_091814.bin", "mod time(min)"=58231651.96666667, "file format"=enum."binary", "power(V)"=2.1, "Magn Field(T) "=0.0}, {"temperature"=14.788, "temperature str"="14.78800", "file path"=path "D:/Data/Ultrasound/LSCO/LSCO22__130814c/5_Cooling_2nd_try/September_2014/091814/14.78800K_500_2500_2.10000V_0.00000T_Sep18-2014__11-33-18_001_091814.bin", 
